vi "Delete Method Template Files.vi"(8 "error in (no error)":errorcluster, 11 "LVClassLibrary in":refnum<vi>) -> (0 "error out":errorcluster, 3 "LVClassLibrary out":refnum<vi>)   [LabVIEW 2019, in "gRPC Template Creation Utility.lvlib"]
uses:
  gRPC Template Creation Utility.lvlib
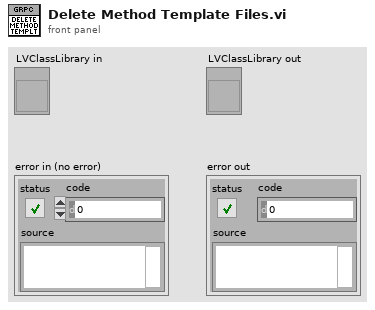
[diagram p1: front panel]
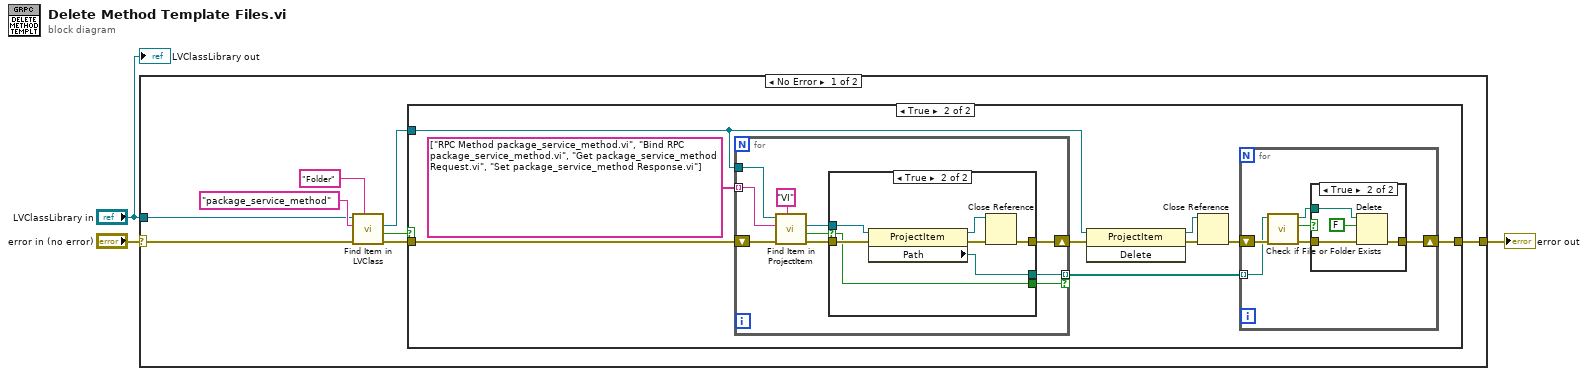
[diagram p0: block diagram]
diagram:
  n1 = case shown="No Error" "error in (no error)" {
    selector: "error in (no error)" -> [w5 w52]
    tunnel: "LVClassLibrary in" -> [w9 _]
    tunnel: [w4 w52] -> w1
    frame No Error {
      n2 = call "Find Item in LVClass.vi"("Item Type"="Folder", "error in (no error)"=w5, "Item Name"="package_service_method", "Class Item in"=w9) -> ("error out"=w7:errorcluster, "Found?"=w6:bool, "Project Item (Class Item)"=w8:refnum<vi>)  [unwired: 4 in, 1 out]
      n3 = case shown="True" w6 {
        tunnel: w8 -> [_ w17]
        tunnel: w7 -> [w12 w21]
        tunnel: [w12 w13] -> w4
        frame False {
        }
        frame True {
          n4 = for {
            tunnel: w17 -> [w42]
            shift-right: [w36] -> w16
            shift-left: w21 -> [w38]
            tunnel: string[] ["RPC Method package_service_method.vi", "Bind RPC package_service_method.vi", "Get package_service_method Request.vi", "Set package_service_method Response.vi"] -> [w35] mode=indexing
            tunnel: [w34] -> w14 mode=indexing if=w33
            n5 = call "Find Item in ProjectItem.vi"("Item Type"="VI", "error in (no error)"=w38, "Name"=w35, "ProjectItem in"=w42) -> ("error out"=w37:errorcluster, "Found ?"=w40:bool, "Item Refnum out"=w39:refnum<vi>)  [unwired: 4 in, 1 out]
            n6 = case shown="True" w40 {
              selector: w40 -> [w43 w45]
              tunnel: w37 -> [w44 w51]
              tunnel: w39 -> [_ w50]
              tunnel: [w44 w46] -> w36
              tunnel: [_ w47] -> w34
              tunnel: [w43 w45] -> w33
              frame False {
              }
              frame True {
                n7 = property class="ProjectItem"(reference=w50, error in=w51) -> (reference out=w49:refnum<vi>, error out=w48:errorcluster, "Path"=w47:path)
                n8 = Close Reference(reference=w49, error in (no error)=w48) -> (error out=w46:errorcluster)
              }
            }
          }
          n9 = invoke class="ProjectItem" method="Delete"(reference=w17, error in=w16) -> (reference out=w18:refnum<vi>, error out=w19:errorcluster)  [unwired: 1 in, 1 out]
          n10 = Close Reference(reference=w18, error in (no error)=w19) -> (error out=w15:errorcluster)
          n11 = for {
            tunnel: w14 -> [w23] mode=indexing
            shift-right: [w22] -> w13
            shift-left: w15 -> [w24]
            n12 = call <vilib>:"Check if File or Folder Exists.vi"("error in (no error)"=w24, "path"=w23) -> ("error out"=w27:errorcluster, "file or folder exists?"=w25:bool, "dup path"=w26:path)  [unwired: 7 in]
            n13 = case shown="True" w25 {
              tunnel: w26 -> [_ w32]
              tunnel: w27 -> [w28 w31]
              tunnel: [w28 w30] -> w22
              frame False {
              }
              frame True {
                n14 = Delete(path (use dialog)=w32, entire hierarchy (F)=FALSE, error in=w31) -> (error out=w30:errorcluster)  [unwired: 2 in, 2 out]
              }
            }
          }
        }
      }
    }
    frame Error {
    }
  }
  "error out" <- w1
  "LVClassLibrary out" <- "LVClassLibrary in"
